vi "Ballard - Arinc-429 - ARINC Channel Page.vi"(8 "error in (no error)":errorcluster, 11 "Node Ptr":T1 format="%.0x") -> (0 "error out":errorcluster)   [LabVIEW 2016, in "Ballard Arinc-429 System Explorer.lvlib"]
uses:
  Ballard Arinc-429 System Explorer.lvlib
  <vilib>/NI VeriStand/Custom Device API/Custom Device API.lvlib
  Shared/Controls and Global/Global.vi
  Shared/Ballard Arinc-429 Shared.lvlib
  <vilib>/NI Veristand/Custom Device API/Get Item Property (U32).vi
  <vilib>/NI Veristand/Custom Device API/Custom Device Item Ref.ctl
panel:
  out "Channel #":u32
  in  "Header":cluster{"Section Name":string}={"Section Name"="Ballard 429 Channel"}
  in  "Description":string
  out "Name":string
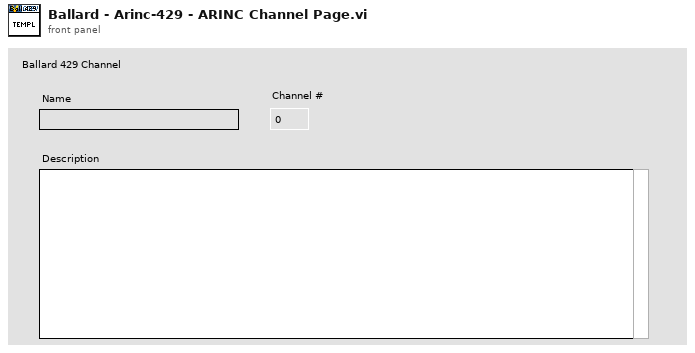
[diagram p1: front panel]
types:
  T1 = typedef "Custom Device API.lvlib/Custom Device Item Ref.ctl" = u64
  T2 = typedef "Custom Device API.lvlib/Custom Device Item Info.ctl" = cluster{"Name":string, "Is Channel":bool, "GUID":string, "Is Waveform":bool}
  T3 = typedef "Custom Device API.lvlib/Custom Device Commands.ctl" = enum16{"Default", "Item renamed", "Shutdown", "Dynamic button pressed"}
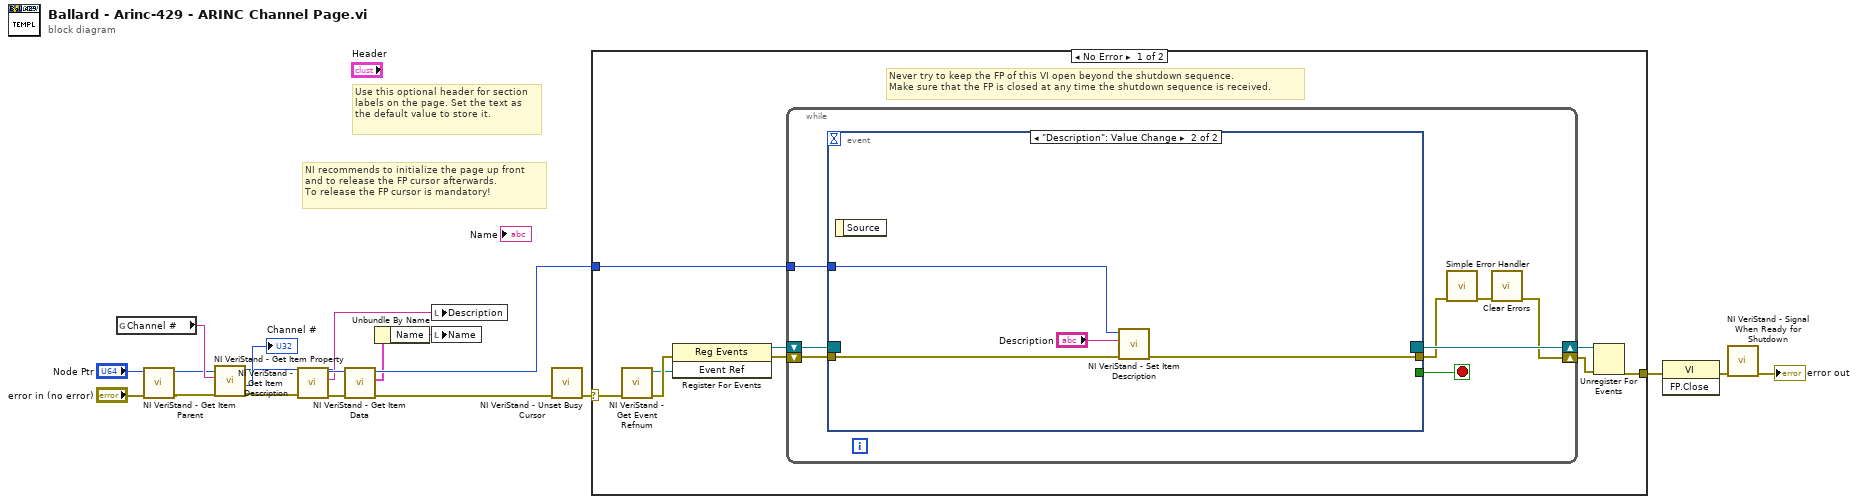
[diagram p0: block diagram]
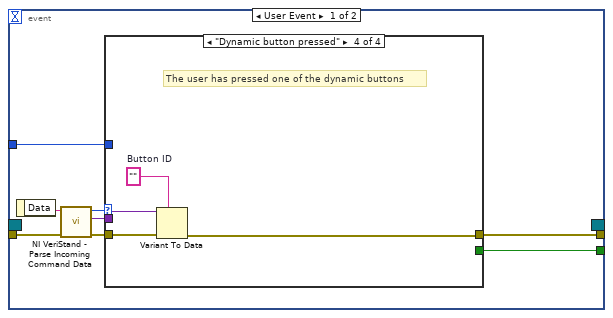
[diagram p2: hidden frame]
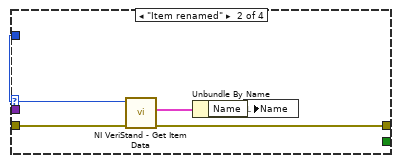
[diagram p4: hidden frame]
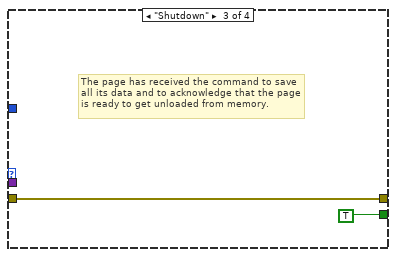
[diagram p5: hidden frame]
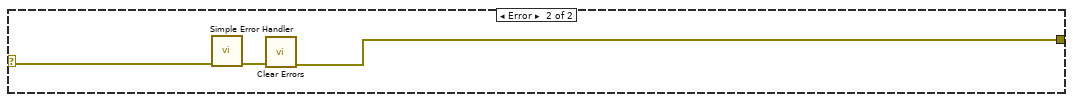
[diagram p6: hidden frame]
diagram:
  # "Use this optional header for section labels on the page. Set the text as the default value to store it."
  # "NI recommends to initialize the page up front\nand to release the FP cursor afterwards.\nTo release the FP cursor is mandatory!"
  n1 = global read "Global.vi" "Channel #"() -> (w8:string)
  n2 = call <vilib>:"NI VeriStand - Get Item Parent.vi"("error in (no error)"="error in (no error)", "Item Ref in"="Node Ptr") -> ("error out"=w1:errorcluster, "Item Ref out"=w4:T1)  [unwired: 6 in, 2 out]
  n3 = call-poly <vilib>:"NI VeriStand - Get Item Property.vi"("error in (no error)"=w1, "Property Name"=w8, "Item Ref in"=w4) -> ("error out"=w3:errorcluster, "Value"=→"Channel #":u32, "Item Ref out"=w2:T1)  [unwired: 5 in, 1 out]
  n4 = call <vilib>:"NI VeriStand - Get Item Description.vi"("error in (no error)"=w3, "Item Ref in"=w2) -> ("error out"=w11:errorcluster, "Description"=w12:string, "Item Ref out"=w13:T1)  [unwired: 7 out]
  n5 = call <vilib>:"NI VeriStand - Get Item Data.vi"("error in (no error)"=w11, "Item Ref in"=w13) -> ("error out"=w16:errorcluster, "Item Info"=w10:T2, "Item Ref out"=w14:T1)  [unwired: 7 out]
  n6 = Unbundle By Name(w10) -> ("Name"=w9:string)
  n7 = local write "Description"(w12) -> ()
  n8 = local write "Name"(w9) -> ()
  n9 = call <vilib>:"NI VeriStand - Unset Busy Cursor.vi"("error in (no error)"=w16) -> ("error out"=w15:errorcluster)  [unwired: 10 out]
  n10 = case shown="No Error" w15 {
    selector: w15 -> [w20 w63]
    tunnel: [w25 w61] -> w19
    tunnel: w14 -> [w21 _]
    frame No Error {
      # "Never try to keep the FP of this VI open beyond the shutdown sequence.\nMake sure that the FP is closed at any time the shutdown sequence is received."
      n11 = call <vilib>:"NI VeriStand - Get Event Refnum.vi"("error in (no error)"=w20) -> ("error out"=w28:errorcluster, "Event Ref"=w24:refnum<user-event>)  [unwired: 9 out]
      n12 = register-events(error in=w28, w24) -> (reference out=w22:refnum<event-registration>, error out=w23:errorcluster)  [unwired: 1 in]
      n13 = while {
        tunnel: w21 -> [w32]
        shift-right: [w29] -> w26
        shift-left: w23 -> [w35]
        shift-right: [w36] -> w27
        shift-left: w22 -> [w34]
        stop <- w33 stop-if-true
        n14 = event shown="[1] \"Description\": Value Change" {
          selector: w34 -> [_ _]
          dyn-events: [_ _] -> w36
          timeout: _ -> [_ _]
          tunnel: w35 -> [w44 w59]
          tunnel: [w40 _] -> w33
          tunnel: [w39 w58] -> w31
          tunnel: w32 -> [w38 w60]
          event User Event {
            n15 = event-data() -> ("Data"=w43:string)  [unwired: 1 out]
            n16 = call <vilib>:"NI VeriStand - Parse Incoming Command Data.vi"("error in (no error)"=w44, "Incoming data"=w43) -> ("error out"=w42:errorcluster, "Outgoing data"=w37:variant, "Action"=w41:T3)  [unwired: 7 out]
            n17 = case shown="\"Dynamic button pressed\"" w41 {
              tunnel: w42 -> [w45 w50 w51 w56]
              tunnel: [_ _ TRUE _] -> w40
              tunnel: [w45 w47 w51 w53] -> w39
              tunnel: w38 -> [_ w49 _ _]
              tunnel: w37 -> [_ _ _ w55]
              frame "Default", Default {
              }
              frame "Item renamed" {
                n18 = call <vilib>:"NI VeriStand - Get Item Data.vi"("error in (no error)"=w50, "Item Ref in"=w49) -> ("error out"=w47:errorcluster, "Item Info"=w48:T2)  [unwired: 8 out]
                n19 = Unbundle By Name(w48) -> ("Name"=w46:string)
                n20 = local write "Name"(w46) -> ()
              }
              frame "Shutdown" {
                # "The page has received the command to save all its data and to acknowledge that the page is ready to get unloaded from memory."
              }
              frame "Dynamic button pressed" {
                w54 = ""  # Button ID
                # "The user has pressed one of the dynamic buttons"
                n21 = Variant To Data(error in=w56, type=w54, Variant=w55) -> (error out=w53:errorcluster)  [unwired: 1 out]
              }
            }
          }
          event "Description": Value Change {
            n22 = event-data() -> ()  [unwired: 2 out]
            n23 = call <vilib>:"NI VeriStand - Set Item Description.vi"("error in (no error)"=w59, "Description"="Description", "Item Ref in"=w60) -> ("error out"=w58:errorcluster)  [unwired: 8 out]
          }
        }
        n24 = call <vilib>:"Simple Error Handler.vi"("error in (no error)"=w31) -> ("error out"=w30:errorcluster)  [unwired: 1 in, 7 out]
        n25 = call <vilib>:"Clear Errors.vi"("error in (no error)"=w30) -> ("error out"=w29:errorcluster)  [unwired: 1 in, 5 out]
      }
      n26 = Unregister For Events(event registration refnum=w27, error in=w26) -> (error out=w25:errorcluster)
    }
    frame Error {
      n27 = call <vilib>:"Simple Error Handler.vi"("error in (no error)"=w63) -> ("error out"=w62:errorcluster)  [unwired: 1 in, 7 out]
      n28 = call <vilib>:"Clear Errors.vi"("error in (no error)"=w62) -> ("error out"=w61:errorcluster)  [unwired: 1 in, 5 out]
    }
  }
  n29 = invoke class="VI" method="FP.Close"(error in=w19) -> (error out=w18:errorcluster)  [unwired: 2 in, 2 out]
  n30 = call <vilib>:"NI VeriStand - Signal When Ready for Shutdown.vi"("error in (no error)"=w18) -> ("error out"=→"error out":errorcluster)  [unwired: 10 out]
